vi "Configure DNS.vi"(0 "VISA resource name":refnum<visa-resource-name>, 1 "Enable Dynamic DNS Registration (T: Enable)":bool=TRUE, 2 "Enable Host Name Verification (T: Enable)":bool=TRUE, 5 "Domain":string, 7 "Host Name (k-26xx)":string="k-26xx", 9 "DNS Address (0.0.0.0)":string="0.0.0.0", 11 "error in (no error)":errorcluster, 12 "DNS Address Index (1)":i32=1) -> (4 "VISA resource name out":refnum<visa-resource-name>, 15 "error out":errorcluster)   [LabVIEW 2019, in "Keithley 2600 Series.lvlib"]
doc: "Configures the basic settings for DNS."
uses:
  Keithley 2600 Series.lvlib
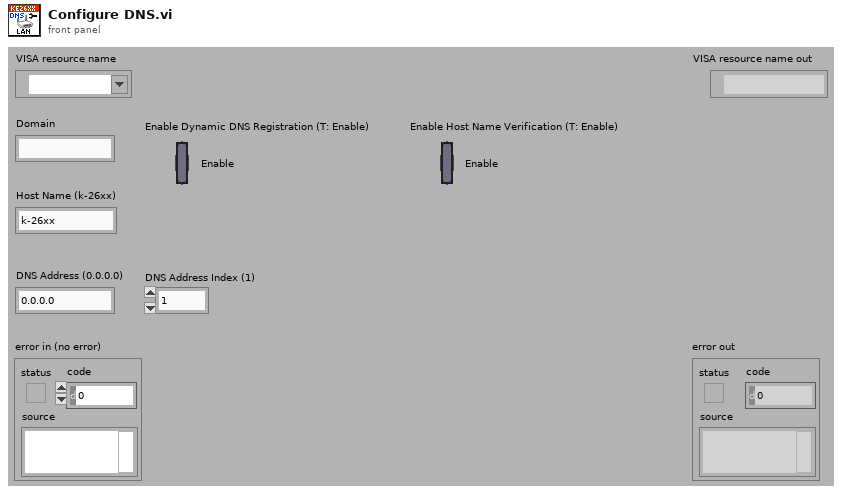
[diagram p1: front panel]
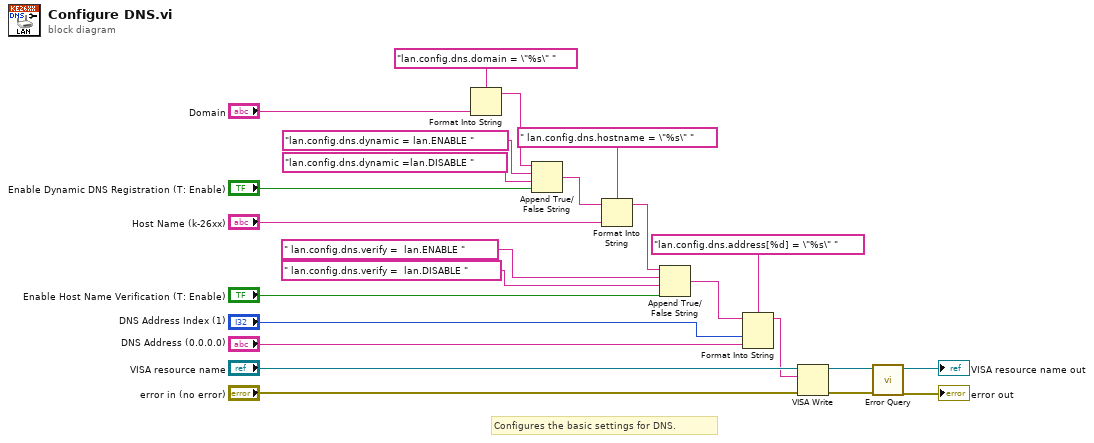
[diagram p0: block diagram]
diagram:
  # "Configures the basic settings for DNS."
  n1 = Format Into String(format string="lan.config.dns.domain = \"%s\" ", "Domain") -> (resulting string=w22:string)  [unwired: 2 in, 1 out]
  n2 = Append True/False String(1:"Enable Dynamic DNS Registration (T: Enable)", 2:"lan.config.dns.dynamic =lan.DISABLE ", 3:"lan.config.dns.dynamic = lan.ENABLE ", 4:w22) -> (0:w18:string)
  n3 = Format Into String(format string=" lan.config.dns.hostname = \"%s\" ", initial string=w18, "Host Name (k-26xx)") -> (resulting string=w15:string)  [unwired: 1 in, 1 out]
  n4 = Append True/False String(1:"Enable Host Name Verification (T: Enable)", 2:" lan.config.dns.verify =  lan.DISABLE ", 3:" lan.config.dns.verify =  lan.ENABLE ", 4:w15) -> (0:w2:string)
  n5 = Format Into String(format string="lan.config.dns.address[%d] = \"%s\" ", initial string=w2, "DNS Address Index (1)", "DNS Address (0.0.0.0)") -> (resulting string=w1:string)  [unwired: 1 in, 1 out]
  n6 = VISA Write(VISA resource name="VISA resource name", write buffer=w1, error in (no error)="error in (no error)") -> (VISA resource name out=w9:refnum<visa-resource-name>, error out=w8:errorcluster)  [unwired: 1 out]
  n7 = call "Error Query.vi"("error in (no error)"=w8, "VISA resource name"=w9) -> ("error out"=→"error out":errorcluster, "VISA resource name out"=→"VISA resource name out":refnum<visa-resource-name>)  [unwired: 6 in, 2 out]
